vi "OPRREADPTR wrapper.vi"(8 "error in (no error)":errorcluster caption="错误输入（无错误）", 9 "pRtnLine":i32, 10 "dwCanNodeId":u32, 11 "dwDevIndex":u32) -> (0 "error out":errorcluster caption="错误输出", 1 "pRtnLine out":i32, 3 "function return":u32)   [LabVIEW 2016, in "UISimCanFunc_wrapper.lvlib"]
doc: "_declspec (dllexport) DWORD OPRREADPTR_wrapper(DWORD dwDevIndex, DWORD dwCanNodeId, PINT pRtnLine);"
uses:
  <userlib>/UISimCanFunc_wrapper/UISimCanFunc_wrapper.lvlib
  <userlib>/UISimCanFunc_wrapper/UISimCanFunc_wrapper.dll
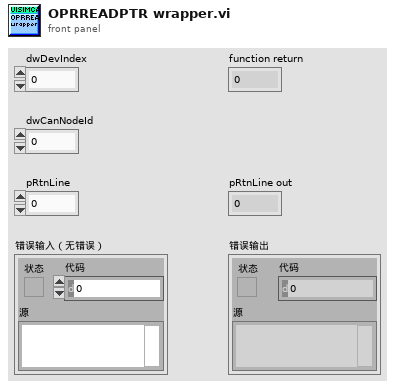
[diagram p1: front panel]
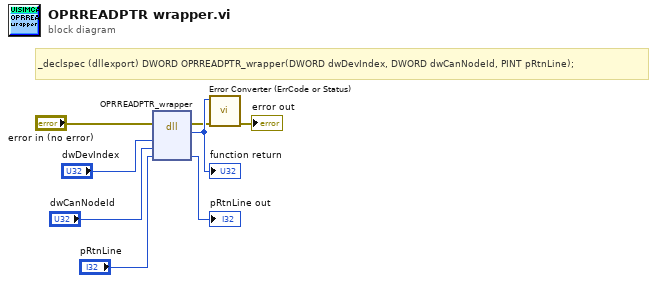
[diagram p0: block diagram]
diagram:
  # "_declspec (dllexport) DWORD OPRREADPTR_wrapper(DWORD dwDevIndex, DWORD dwCanNodeId, PINT pRtnLine);"
  n1 = dll-call lib="C:/Program Files (x86)/National Instruments/LabVIEW 2016/user.lib/UISimCanFunc_wrapper/UISimCanFunc_wrapper.*" fn="OPRREADPTR_wrapper"(error in="error in (no error)", "dwDevIndex"="dwDevIndex", "dwCanNodeId"="dwCanNodeId", "pRtnLine"="pRtnLine") -> (error out=w2:errorcluster, w8:u32, "pRtnLine"=→"pRtnLine out":i32)  [unwired: 4 in, 1 out]
  "function return" <- w8
  n2 = call <userlib>:"Error Converter (ErrCode or Status).vi"("error in (no error)"=w2, "error code"=w8) -> ("error out"=→"error out":errorcluster)  [unwired: 9 in]
